vi "check Abort (ActiveJob).vi"(8 "error in (no error)":errorcluster, 9 "timeout (0 ms)":i32, 11 "Job in":refnum<class "Job.lvclass">) -> (0 "error out":errorcluster, 1 "exception":i32, 2 "Abort":bool, 3 "Job out":refnum<class "Job.lvclass">)   [LabVIEW 2013, in "openCronJob.lvlib" / "Job.lvclass"]
uses:
  Job.lvclass
  Job.lvclass/Job.ctl
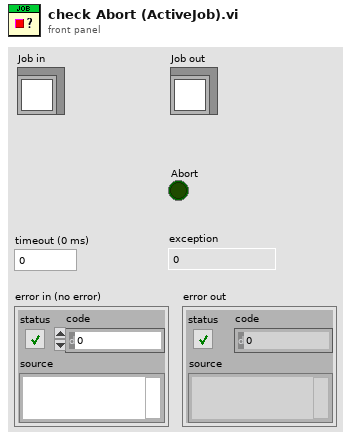
[diagram p1: front panel]
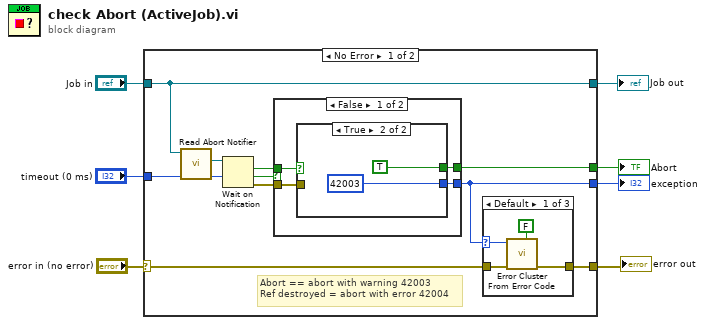
[diagram p0: block diagram]
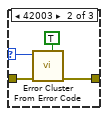
[diagram p2: hidden frame]
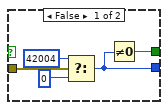
[diagram p4: hidden frame]
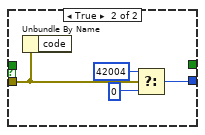
[diagram p5: hidden frame]
diagram:
  n1 = case shown="No Error" "error in (no error)" {
    selector: "error in (no error)" -> [w8 w43]
    tunnel: [w17 _] -> w7
    tunnel: [w10 _] -> w6
    tunnel: "timeout (0 ms)" -> [w14 _]
    tunnel: "Job in" -> [w11 w42]
    tunnel: [w11 w42] -> w2
    tunnel: [w9 w43] -> w1
    frame No Error {
      # "Abort == abort with warning 42003\nRef destroyed = abort with error 42004"
      n2 = call "Read Abort Notifier.vi"("Job in"=w11) -> ("Abort"=w13:refnum<notifier>)  [unwired: 10 in]
      n3 = Wait on Notification(notifier=w13, timeout in ms (-1)=w14) -> (notification=w15:bool, timed out?=w12:bool, error out=w16:errorcluster)  [unwired: 2 in, 1 out]
      n4 = case shown="False" w12 {
        tunnel: [w30 _] -> w17
        tunnel: w16 -> [w29 w38]
        tunnel: w15 -> [w28 _]
        tunnel: [w27 w39] -> w10
        frame False {
          n5 = case shown="True" w28 {
            tunnel: [w31 42003 ("exception")] -> w27
            tunnel: w29 -> [w35 _]
            tunnel: [w32 TRUE] -> w30
            frame False {
              n6 = Select(t=42004, s=w35, f=0 ("exception")) -> (s? t:f=w31:i32)
              n7 = Not Equal To 0?(x=w31) -> (x != 0?=w32:bool)
            }
            frame True {
            }
          }
        }
        frame True {
          n8 = Unbundle By Name(w38) -> ()  [unwired: 1 out]
          n9 = Select(t=42004, s=w38, f=0 ("exception")) -> (s? t:f=w39:i32)
        }
      }
      n10 = case shown="Default" w10 {
        selector: w10 -> [w19 w23 _]
        tunnel: [w20 w24 w26] -> w9
        tunnel: w8 -> [w21 w25 w26]
        frame Default {
          n11 = call <vilib>:"Error Cluster From Error Code.vi"("is warning? (False)"=FALSE, "error in (no error)"=w21, "error code (0)"=w19) -> ("error out"=w20:errorcluster)  [unwired: 6 in]
        }
        frame 42003 {
          n12 = call <vilib>:"Error Cluster From Error Code.vi"("is warning? (False)"=TRUE, "error in (no error)"=w25, "error code (0)"=w23) -> ("error out"=w24:errorcluster)  [unwired: 6 in]
        }
        frame 0 {
        }
      }
    }
    frame Error {
    }
  }
  "Abort" <- w7
  "exception" <- w6
  "Job out" <- w2
  "error out" <- w1
